vi "XY Graph Get TipStrip Refnum.vi"(8 "Error In":errorcluster, 11 "XYGraph Refnum":T1) -> (0 "Error Out":errorcluster, 1 "TipStrip Refnum Found?":bool, 2 "TipStrip Refnum":refnum<vi>, 3 "XYGraph Refnum":T1)   [LabVIEW 2021, in "XY Graph Add-Ons.lvlib"]
uses:
  XY Graph Add-Ons.lvlib
  XY Graph Refnum.ctl
  Utilities/Utilities.lvlib
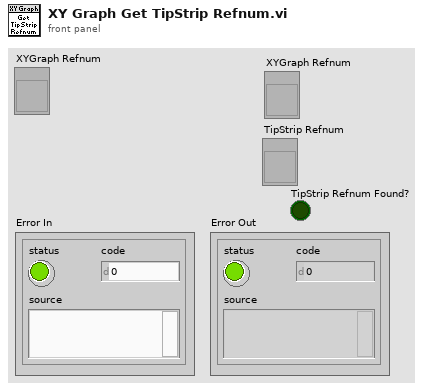
[diagram p1: front panel]
types:
  T1 = typedef "XY Graph Add-Ons.lvlib/XY Graph Refnum.ctl" = refnum<vi>
  T2 = enum16{"Controls & Indicators", "Controls", "Indicators"}
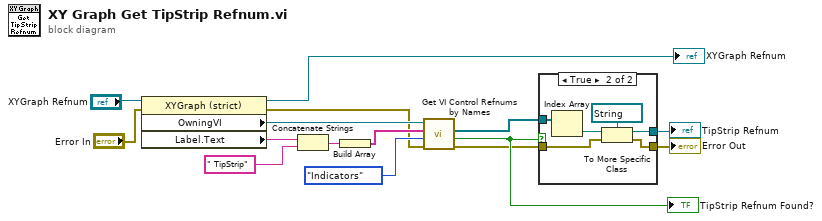
[diagram p0: block diagram]
diagram:
  n1 = property class="XYGraph (strict)"(reference="XYGraph Refnum", error in="Error In") -> (reference out=→"XYGraph Refnum":T1, error out=w8:errorcluster, "OwningVI"=w12:refnum<vi>, "Label.Text"=w13:string)
  n2 = Concatenate Strings(w13, " TipStrip" ("string")) -> (w11:string)
  n3 = Build Array(w11) -> (w10:string[])
  n4 = call "Get VI Control Refnums by Names.vi"("error in"=w8, "Selection"=T2."Indicators", "Control Labels"=w10, "VI  Ref"=w12) -> ("error out"=w1:errorcluster, "All Ctls found?"=w3:bool, "Ctl Refnums"=w7:refnum<vi>[])  [unwired: 4 in, 1 out]
  "TipStrip Refnum Found?" <- w3
  n5 = case shown="True" w3 {
    tunnel: w7 -> [_ w22]
    tunnel: [_ w20] -> w6
    tunnel: w1 -> [w16 w19]
    tunnel: [w16 w17] -> w4
    frame False {
    }
    frame True {
      n6 = Index Array(array=w22) -> (element=w21:refnum<vi>)  [unwired: 1 in]
      n7 = To More Specific Class(target class=refnum<vi> refnum ("TipStrip Refnum"), reference=w21, error in=w19) -> (specific class reference=w20:refnum<vi>, error out=w17:errorcluster)
    }
  }
  "TipStrip Refnum" <- w6
  "Error Out" <- w4
